vi "ADCP_UI_Queues_FGV.vi"(2 "error in (no error)":errorcluster, 3 "Initialize ?":bool) -> (0 "error out":errorcluster, 1 "Queues":T1)   [LabVIEW 2017]
uses:
  Controls/ADCP_UI/ADCP_UI_Queues.ctl
  Controls/ADCP_UI/ADCP_UI_Continuous_Receiver_States.ctl
  Controls/ADCP_UI/ADCP_Queue_Receive_Log_Queue_Element.ctl
  Controls/Packet/Packet.ctl
  Controls/Packet/Packet_Direction.ctl
  Controls/Packet/Packet_Type.ctl
  Controls/Packet/Packet_Priority.ctl
  Controls/Data Packets/Data_Packet.ctl
  Controls/Data Packets/Parameter.ctl
  Controls/Data Packets/Parameter_Data_Type.ctl
  Controls/Data Packets/Data_Packet_Transmit_Mode.ctl
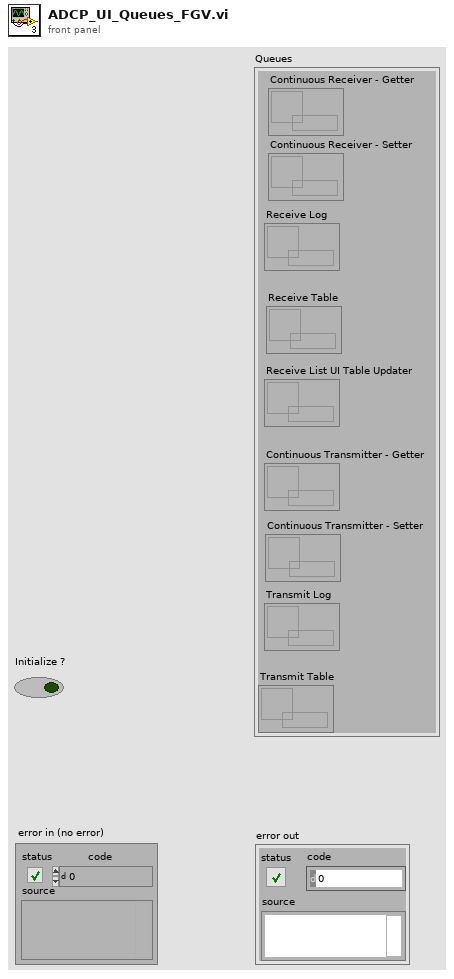
[diagram p1: front panel]
types:
  T1 = typedef "ADCP_UI_Queues.ctl" = cluster{"Continuous Receiver - Getter":refnum<queue>, "Continuous Receiver - Setter":refnum<queue>, "Receive Log":refnum<queue>, "Receive Table":refnum<queue>, "Receive List UI Table Updater":refnum<queue>, "Continuous Transmitter - Getter":refnum<queue>, "Continuous Transmitter - Setter":refnum<queue>, "Transmit Log":refnum<queue>, "Transmit Table":refnum<queue>}
  T2 = typedef "Data_Packet.ctl" = cluster{"Packet":T3, "Parameters":T7[], "Last Received Time (ms)":u64, "Receive count":i32, "Transmit count":i32, "Transmit interval (ms)":u32, "Last Transmitted Time (ms)":u64, "Receive interval (ms)":u32, "Transmit_Mode":T9, "Transmit Enable":bool, "Cyclic Transmit interval (ms)":u32}
  T3 = typedef "Packet.ctl" = cluster{"Raw Bytes":u8[], "Checksum":bool, "Direction":T4, "Processed Bytes":u8[], "Node ID":u8, "Packet type":T5, "Frame Data":u32, "Priority":T6, "Frame ID":u8}
  T4 = typedef "Packet_Direction.ctl" = enum16{"Transmit", "Receive", "Bidirectional"}
  T5 = typedef "Packet_Type.ctl" = enum16{"Data", "Connection Management", "Remote Request", "Error/Status"}
  T6 = typedef "Packet_Priority.ctl" = enum16{"LOW", "HIGH"}
  T7 = typedef "Parameter.ctl" = cluster{"Parameter name":string, "Node name":string, "Node ID":u8, "Frame name":string, "Frame ID":u8, "Data type":T8, "Start Bit":i32, "Bit Length":i32, "Factor":dbl, "Offset":dbl, "Minimum":dbl, "Maximum":dbl, "Descriptor":string, "Enum values":string[], "Value":string}
  T8 = typedef "Parameter_Data_Type.ctl" = enum16{"BOOL", "UNSIGNED", "SIGNED", "FLOAT32", "ENUM"}
  T9 = typedef "Data_Packet_Transmit_Mode.ctl" = enum16{"Disabled", "Single", "Cyclic"}
  T10 = typedef "ADCP_Queue_Receive_Log_Queue_Element.ctl" = cluster{"Packet":T3, "Receive Time (ms)":u64, "Count":i32, "Receive Time Interval (ms) ":u64}
  T11 = typedef "ADCP_UI_Continuous_Receiver_States.ctl" = enum16{"Disable", "Enable", "Exit"}
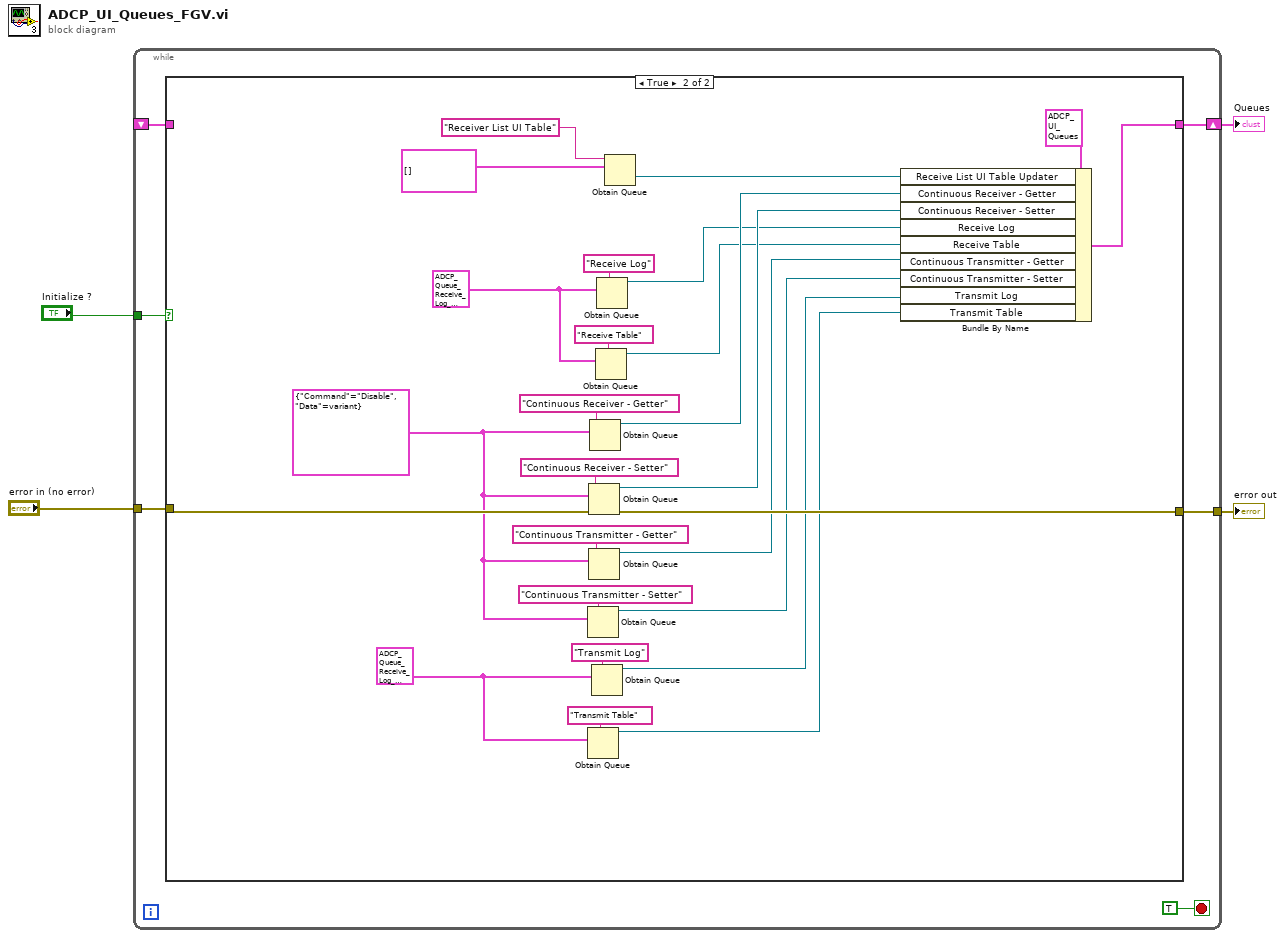
[diagram p0: block diagram]
diagram:
  n1 = while {
    tunnel: "Initialize ?" -> [w9]
    tunnel: "error in (no error)" -> [w8]
    tunnel: [w7] -> w1
    shift-right: [w6] -> w2
    shift-left: _ -> [w5]
    stop <- TRUE stop-if-true
    n2 = case shown="True" w9 {
      tunnel: w8 -> [w11 w36]
      tunnel: [w11 w35] -> w7
      tunnel: [w12 w31] -> w6
      tunnel: w5 -> [w12 _]
      frame False {
      }
      frame True {
        w17 = T10 {"Packet"={"Raw Bytes"=[], "Checksum"=FALSE, "Direction"=enum."Transmit", "Processed Bytes"=[], "Node ID"=0, "Packet type"=enum."Data", "Frame Data"=0, "Priority"=enum."LOW", "Frame ID"=0}, "Receive Time (ms)"=0, "Count"=0, "Receive Time Interval (ms) "=0}
        w28 = T10 {"Packet"={"Raw Bytes"=[], "Checksum"=FALSE, "Direction"=enum."Transmit", "Processed Bytes"=[], "Node ID"=0, "Packet type"=enum."Data", "Frame Data"=0, "Priority"=enum."LOW", "Frame ID"=0}, "Receive Time (ms)"=0, "Count"=0, "Receive Time Interval (ms) "=0}
        w20 = cluster{"Command":T11, "Data":variant} {"Command"=enum."Disable", "Data"=variant}
        n3 = Obtain Queue(name (unnamed)="Continuous Transmitter - Setter", element data type=w20) -> (queue out=w15:refnum<queue>)  [unwired: 3 in, 2 out]
        n4 = Obtain Queue(name (unnamed)="Transmit Table", element data type=w17) -> (queue out=w13:refnum<queue>)  [unwired: 3 in, 2 out]
        n5 = Obtain Queue(name (unnamed)="Continuous Receiver - Setter", element data type=w20, error in (no error)=w36) -> (queue out=w32:refnum<queue>, error out=w35:errorcluster)  [unwired: 2 in, 1 out]
        n6 = Obtain Queue(name (unnamed)="Continuous Transmitter - Getter", element data type=w20) -> (queue out=w16:refnum<queue>)  [unwired: 3 in, 2 out]
        n7 = Obtain Queue(name (unnamed)="Continuous Receiver - Getter", element data type=w20) -> (queue out=w33:refnum<queue>)  [unwired: 3 in, 2 out]
        n8 = Obtain Queue(name (unnamed)="Transmit Log", element data type=w17) -> (queue out=w14:refnum<queue>)  [unwired: 3 in, 2 out]
        n9 = Obtain Queue(name (unnamed)="Receive Table", element data type=w28) -> (queue out=w26:refnum<queue>)  [unwired: 3 in, 2 out]
        n10 = Obtain Queue(name (unnamed)="Receive Log", element data type=w28) -> (queue out=w27:refnum<queue>)  [unwired: 3 in, 2 out]
        n11 = Obtain Queue(name (unnamed)="Receiver List UI Table", element data type=T2[] []) -> (queue out=w23:refnum<queue>)  [unwired: 3 in, 2 out]
        n12 = Bundle By Name(cluster=T1 {"Continuous Receiver - Getter"=refnum, "Continuous Receiver - Setter"=refnum, "Receive Log"=refnum, "Receive Table"=refnum, "Receive List UI Table Updater"=refnum, "Continuous Transmitter - Getter"=refnum, "Continuous Transmitter - Setter"=refnum, "Transmit Log"=refnum, "Transmit Table"=refnum} ("Cluster"), "Receive List UI Table Updater"=w23, "Continuous Receiver - Getter"=w33, "Continuous Receiver - Setter"=w32, "Receive Log"=w27, "Receive Table"=w26, "Continuous Transmitter - Getter"=w16, "Continuous Transmitter - Setter"=w15, "Transmit Log"=w14, "Transmit Table"=w13) -> (w31:T1)
      }
    }
  }
  "Queues" <- w2
  "error out" <- w1
